vi "Request Message.vi"(4 "Ignore Past Updates? (F)":bool, 5 "Return Priority (Normal)":T1=enum."Normal", 6 "Value Changes Only? (T)":bool=TRUE, 7 "Notification Msg (Type)":refnum<class "Notification Msg.lvclass">, 8 "error in (no error)":errorcluster, 9 "Data Type":variant, 10 "Datum Name":string, 11 "IObserver in":refnum<class "IObserver.lvclass">) -> (0 "error out":errorcluster, 3 "IObserver out":refnum<class "IObserver.lvclass">)   [LabVIEW 2015, in "IObserver.lvlib" / "IObserver.lvclass"]
doc: "<License>\nCopyright © 2017 Composed Systems, LLC | All rights reserved\nwww.composed.io\n\nAuthor: Ethan Stern <ethan.stern@composed.io>\n\nThis software is provided \"AS IS\" WITHOUT WARRANTIES, either express or implied, AND IS FOR EDUCATIONAL PURPOSES ONLY.\n</License>"
uses:
  IObserver.lvclass
  Transport/ActorMessage/Notification Msg/Notification Msg.lvclass
  <vilib>/ActorFramework/Message Enqueuer/Message Priority.ctl
  <vilib>/ActorFramework/Actor/Actor.lvclass/Actor.ctl
  <vilib>/ActorFramework/Message Enqueuer/Message Enqueuer.lvclass/Message Enqueuer.ctl
  SubscriptionPolicy/BasicSubscription/BasicSubscription.lvclass/BasicSubscription.ctl
  SubscriptionPolicy/ValueChangeSubscription/ValueChangeSubscription.lvclass/ValueChangeSubscription.ctl
  IObserver Messages/Subscribe Msg/Subscribe Msg.lvclass/Subscribe Msg.ctl
  <vilib>/ActorFramework/Message Enqueuer/Init from Existing Queue.vi
  <vilib>/ActorFramework/Message Enqueuer/Enqueue.vi
  <vilib>/ActorFramework/Message Priority Queue/Priority Enqueue.vi
  <vilib>/ActorFramework/Message Enqueuer/Message Enqueuer.lvclass
  SubscriptionPolicy/BasicSubscription/BasicSubscription.lvclass
  SubscriptionPolicy/ValueChangeSubscription/ValueChangeSubscription.lvclass
  IObserver Messages/Subscribe Msg/Subscribe Msg.lvclass
  IMediator/SubscriptionRequest/SubscriptionRequest.lvclass
  <vilib>/ActorFramework/Actor/Actor.lvclass
  Transport/ActorMessage/ActorMessage.lvclass
  IMediator/ISubscriptionPolicy/ISubscriptionPolicy.lvclass
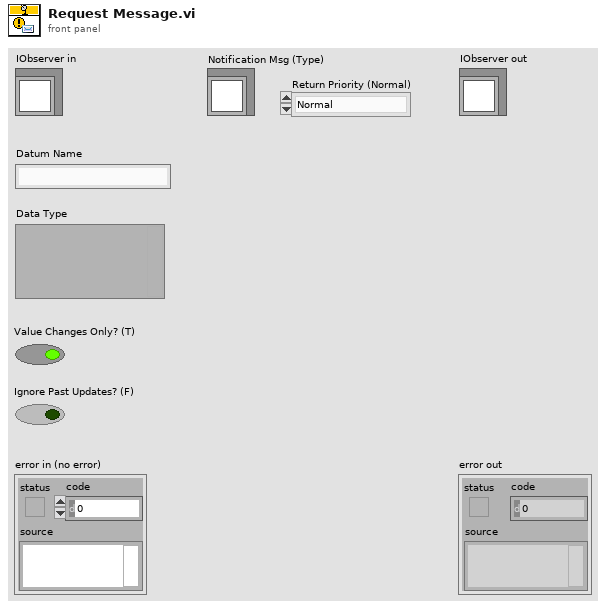
[diagram p1: front panel]
types:
  T1 = typedef "Actor Framework.lvlib/Message Enqueuer.lvclass/Message Priority.ctl" = enum16{"Low", "Normal", "High"}
  T2 = typedef "IMediator.lvlib/ISubscriptionPolicy.lvclass/ISubscriptionPolicy Reference.ctl" = refnum<data-value>
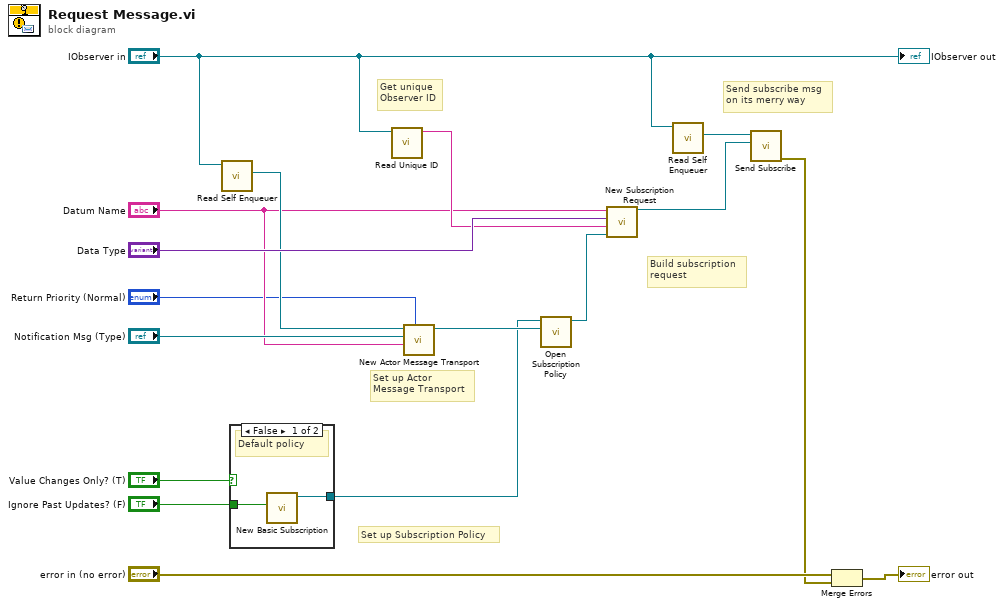
[diagram p0: block diagram]
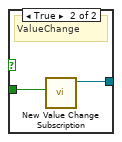
[diagram p2: hidden frame]
diagram:
  # "Set up Subscription Policy"
  # "Send subscribe msg\non its merry way"
  # "Build subscription\nrequest"
  # "Get unique\nObserver ID"
  # "Set up Actor\nMessage Transport"
  n1 = call <vilib>:"Read Self Enqueuer.vi"("Actor"="IObserver in") -> ("Self Enqueuer"=w4:refnum<class "Message Enqueuer.lvclass">)  [unwired: 10 in]
  n2 = case shown="False" "Value Changes Only? (T)" {
    tunnel: "Ignore Past Updates? (F)" -> [w18 w21]
    tunnel: [w19 w20] -> w5
    frame False {
      # "Default policy"
      n3 = call "New Basic Subscription.vi"("Ignore Past Updates? (F)"=w18) -> ("BasicSubscription Out"=w19:refnum<class "BasicSubscription.lvclass">)  [unwired: 10 in]
    }
    frame True {
      # "ValueChange"
      n4 = call "New Value Change Subscription.vi"("Ignore Past Updates? (F)"=w21) -> ("ValueChangeSubscription Out"=w20:refnum<class "ValueChangeSubscription.lvclass">)  [unwired: 10 in]
    }
  }
  n5 = call "Read Unique ID.vi"("IObserver In"="IObserver in") -> ("Unique ID"=w10:string)  [unwired: 10 in]
  n6 = call "New Actor Message Transport.vi"("Return Priority (Normal)"="Return Priority (Normal)", "Datum Name"="Datum Name", "Desired Notification Msg (Type)"="Notification Msg (Type)", "Message Enqueuer in"=w4) -> ("ActorMessage out"=w8:refnum<class "ActorMessage.lvclass">)  [unwired: 6 in, 1 out]
  n7 = call "Open Subscription Policy.vi"("Transport"=w8, "SubscriptionPolicy"=w5) -> ("Subscription Policy"=w9:T2)  [unwired: 8 in, 1 out]
  n8 = call "New Subscription Request.vi"("Subscription Policy"=w9, "Unique Subscriber ID"=w10, "Type"="Data Type", "Datum Name"="Datum Name") -> ("SubscriptionRequest"=w15:refnum<class "SubscriptionRequest.lvclass">)  [unwired: 7 in]
  n9 = call <vilib>:"Read Self Enqueuer.vi"("Actor"="IObserver in") -> ("Self Enqueuer"=w16:refnum<class "Message Enqueuer.lvclass">)  [unwired: 10 in]
  n10 = call "Send Subscribe.vi"("SubscriptionRequest"=w15, "Message Enqueuer"=w16) -> ("error out"=w13:errorcluster)  [unwired: 8 in, 1 out]
  n11 = Merge Errors("error in (no error)", w13) -> (→"error out":errorcluster)
  "IObserver out" <- "IObserver in"
